vi "Install all from repository.vi"(7 "restart automatically (T)":bool=TRUE, 8 "error in (no error)":errorcluster, 10 "Repository Location":string, 11 "RT Management in":refnum<class "RT Management.lvclass">) -> (0 "error out":errorcluster, 3 "RT Management out":refnum<class "RT Management.lvclass">)   [LabVIEW 2016, in "RT Management.lvlib" / "RT Management.lvclass"]
doc: "Installs the latest software versions from the given repository. For PXI systems, this installs all available components, and for cRIO systems, this installs the latest RSS plus all addons minus a few addons. View the addon blacklist in \"RSS addons blacklist.vi\"."
uses:
  RT Management.lvclass
  <vilib>/nisyscfg/Broken Dependency 1.2.ctl
  <vilib>/nisyscfg/Software 1.2.ctl
  <vilib>/nisyscfg/Component Type.ctl
  RT Management.lvclass/RT Management.ctl
  Get SysCfg Session.vi
  <vilib>/nisyscfg/Install All.vi
  <resource>/objmgr/nisysapi.rc
  <vilib>/nisyscfg/nisyscfg.lvlib
panel:
  out "broken dependencies":T1[](array[typedef]) {"dependee"."component type" items=["standard", "hidden", "system", "unknown", "startup"]; "depender"."component type" items=["standard", "hidden", "system", "unknown", "startup"]}
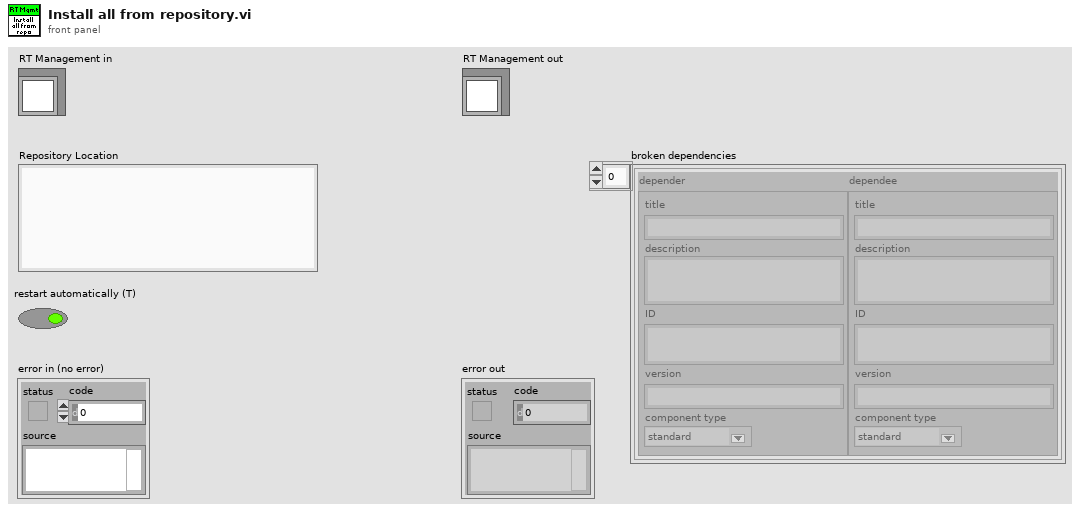
[diagram p1: front panel]
types:
  T1 = typedef "nisyscfg.lvlib/Broken Dependency 1.2.ctl" = cluster{"depender":T2, "dependee":T2}
  T2 = typedef "nisyscfg.lvlib/Software 1.2.ctl" = cluster{"title":string, "description":string, "ID":string, "version":string, "component type":T3}
  T3 = typedef "nisyscfg.lvlib/Component Type.ctl" = u32
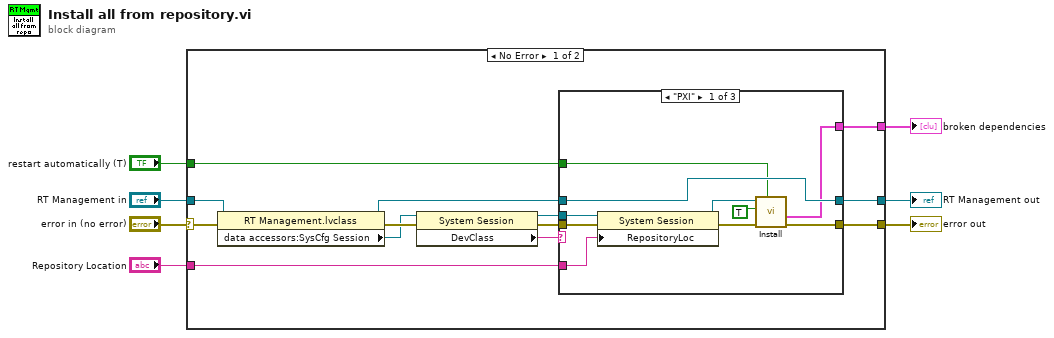
[diagram p0: block diagram]
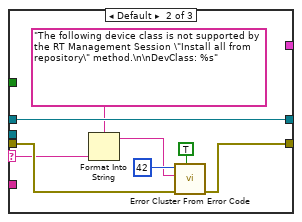
[diagram p2: hidden frame]
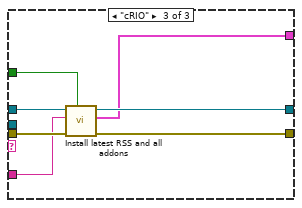
[diagram p3: hidden frame]
diagram:
  n1 = case shown="No Error" "error in (no error)" {
    selector: "error in (no error)" -> [w14 w47]
    tunnel: [w11 w47] -> w6
    tunnel: [w15 w46] -> w4
    tunnel: "RT Management in" -> [w19 w46]
    tunnel: "Repository Location" -> [w12 _]
    tunnel: "restart automatically (T)" -> [w9 _]
    tunnel: [w8 _] -> w1
    frame No Error {
      n2 = property class="RT Management.lvclass"(reference=w19, error in=w14) -> (reference out=w13:refnum<class "RT Management.lvclass">, error out=w20:errorcluster, "data accessors:SysCfg Session"=w18:refnum<k21>)
      n3 = property class="System Session"(reference=w18, error in=w20) -> (reference out=w10:refnum<k21>, error out=w16:errorcluster, "DevClass"=w17:string)
      n4 = case shown="\"PXI\"" w17 {
        selector: w17 -> [_ w34 _]
        tunnel: w16 -> [w30 w38 w45]
        tunnel: [w23 w36 w44] -> w15
        tunnel: w13 -> [w23 w36 w43]
        tunnel: w12 -> [w28 _ w41]
        tunnel: [w24 w37 w42] -> w11
        tunnel: w10 -> [w29 _ _]
        tunnel: w9 -> [w22 _ w40]
        tunnel: [w21 _ w39] -> w8
        frame "PXI" {
          n5 = property class="System Session"(reference=w29, error in=w30, "RepositoryLoc"=w28) -> (reference out=w26:refnum<k21>, error out=w27:errorcluster)
          n6 = call-poly <vilib>:"Install.vi"("Restart Automatically (T)"=w22, "error in (no error)"=w27, "Deselect Conflicts (F)"=TRUE ("deselect conflicts (F)"), "Session in"=w26) -> ("error out"=w24:errorcluster, "Broken Dependencies"=w21:T1[])  [unwired: 4 in, 2 out]
        }
        frame Default {
          n7 = Format Into String(format string="The following device class is not supported by the RT Management Session \"Install all from repository\" method.\n\nDevClass: %s" ("error message (\"\")"), w34) -> (resulting string=w33:string)  [unwired: 2 in, 1 out]
          n8 = call <vilib>:"Error Cluster From Error Code.vi"("show call chain? (False)"=TRUE, "error in (no error)"=w38, "error message (\"\")"=w33, "error code (0)"=42) -> ("error out"=w37:errorcluster)  [unwired: 5 in]
        }
        frame "cRIO" {
          n9 = call "Install latest RSS and all addons.vi"("restart automatically (T)"=w40, "error in (no error)"=w45, "Repository Location"=w41, "RT Management in"=w43) -> ("error out"=w42:errorcluster, "broken dependencies"=w39:T1[], "RT Management out"=w44:refnum<class "RT Management.lvclass">)  [unwired: 5 in]
        }
      }
    }
    frame Error {
    }
  }
  "error out" <- w6
  "RT Management out" <- w4
  "broken dependencies" <- w1
